vi "Delete.vi"(8 "error in (no error)":errorcluster, 11 "Test Configs In":T1) -> (0 "error out":errorcluster, 3 "Test Configs Out":T1)   [LabVIEW 2015]
doc: "Remove the current element from the array of sequence parameters."
uses:
  Type Defs/Sequence Parameters Ref.ctl
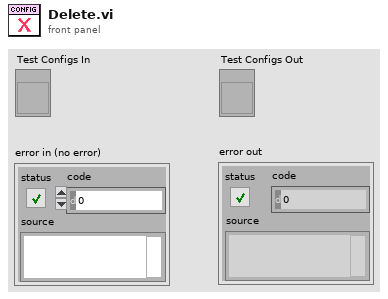
[diagram p1: front panel]
types:
  T1 = typedef "Sequence Parameters Ref.ctl" = refnum<vi>
  T2 = typedef "Sequence Parameters.ctl" = cluster{"Test Name":string, "Target":T3, "Host IP Address":string, "Target IP Address":string, "Shared Variable Host":enum16{"Target", "Host"}, "Shared Variable Writer":enum16{"Target", "Host"}, "Variable Data Type":T4, "# of Variables per Library":u16, "Update Rate (Hz)":dbl, "Read Rate (Hz)":dbl, "Floor":u32, "Ceiling":u32, "Delta":u32}
  T3 = typedef "Target Type.ctl" = enum16{"cRIO-9012", "cRIO-9014", "cRIO-9022", "cRIO-9023", "cRIO-9024", "cRIO-9025", "cRIO-9068", "cRIO-9073", "cRIO-9074", "cRIO-9075", "cRIO-9076", "cRIO-9081", "cRIO-9082", "myRIO-1900", "myRIO-1950", "PXI-8101", "PXI-8115", "PXI-8119", "PXI-8820", "PXIe-8100", "PXIe-8101", "PXIe-8133", "PXIe-8135", "PXIe-8820", "sbRIO-9605", "sbRIO-9606", "sbRIO-9623", "sbRIO-9626", "sbRIO-9633", "sbRIO-9636", "Unlisted (Linux-RT)", "Unlisted (PharLap)", "Unlisted (VxWorks)", "Windows Target"}
  T4 = typedef "Variable Data Type.ctl" = enum16{"U8", "U16", "U32", "U64", "I8", "I16", "I32", "I64", "Single", "Double", "Boolean", "String"}
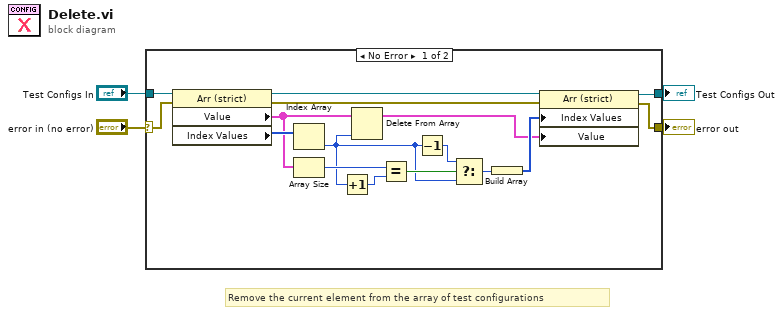
[diagram p0: block diagram]
diagram:
  # "Remove the current element from the array of test configurations"
  n1 = case shown="No Error" "error in (no error)" {
    selector: "error in (no error)" -> [w19 w21]
    tunnel: "Test Configs In" -> [w20 w22]
    tunnel: [w15 w22] -> w1
    tunnel: [w14 w21] -> w3
    frame No Error {
      n2 = property class="Arr (strict)"(reference=w20, error in=w19) -> (reference out=w17:T1, error out=w16:errorcluster, "Value"=w13:T2[], "Index Values"=w18:u32[])
      n3 = Index Array(array=w18) -> (element=w8:u32)  [unwired: 1 in]
      n4 = Array Size(array=w13) -> (size(s)=w12:i32)
      n5 = Increment(x=w8) -> (x+1=w11:u32)
      n6 = Delete From Array(array=w13, index=w8) -> (array with subset deleted=w5:T2[])  [unwired: 1 in, 1 out]
      n7 = Equal?(x=w12, y=w11) -> (x = y?=w10:bool)
      n8 = Decrement(x=w8) -> (x-1=w9:u32)
      n9 = Select(t=w9, s=w10, f=w8) -> (s? t:f=w7:u32)
      n10 = Build Array(w7) -> (w6:u32[])
      n11 = property class="Arr (strict)"(reference=w17, error in=w16, "Index Values"=w6, "Value"=w5) -> (reference out=w15:T1, error out=w14:errorcluster)
    }
    frame Error {
    }
  }
  "error out" <- w3
  "Test Configs Out" <- w1
